vi "get_daq_resources.vi"(8 "error in (no error)":errorcluster) -> (0 "error out":errorcluster, 2 "Resources out":refnum<k20>[](array[refnum]), 3 "Refnum out":refnum<k21>)   [LabVIEW 2015]
uses:
  <vilib>/nisyscfg/nisyscfg.lvlib
  <resource>/objmgr/nisysapi.rc
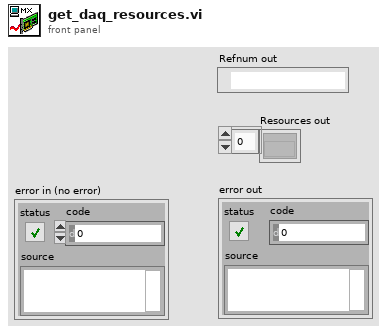
[diagram p1: front panel]
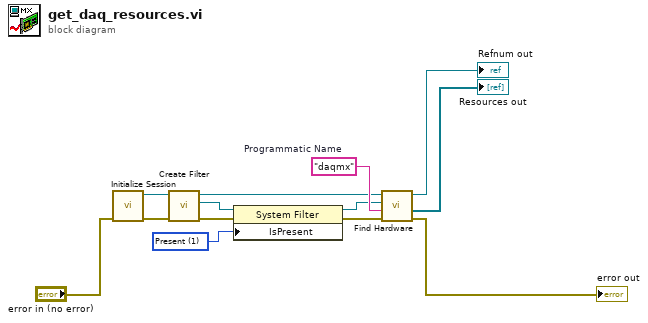
[diagram p0: block diagram]
diagram:
  w4 = 1 items=["Unknown"=-1, "Not Present"=0, "Present"=1] ("Is Present")
  w11 = "daqmx"  # Programmatic Name
  n1 = call <vilib>:"Initialize Session.vi"("error in (no error)"="error in (no error)") -> ("error out"=w2:errorcluster, "Session out"=w3:refnum<k21>)  [unwired: 9 in]
  n2 = call <vilib>:"Create Filter.vi"("error in (no error)"=w2, "Session in"=w3) -> ("error out"=w7:errorcluster, "Filter out"=w8:refnum<k20>, "Session out"=w1:refnum<k21>)  [unwired: 7 in]
  n3 = property class="System Filter"(reference=w8, error in=w7, "IsPresent"=w4) -> (reference out=w5:refnum<k20>, error out=w6:errorcluster)
  n4 = call <vilib>:"Find Hardware.vi"("error in (no error)"=w6, "Experts"=w11, "Filter in"=w5, "Session in"=w1) -> ("error out"=→"error out":errorcluster, "Resources out"=→"Resources out":refnum<k20>[], "Session out"=→"Refnum out":refnum<k21>)  [unwired: 4 in, 1 out]
